vi "Begin.vi"() -> (0 "error out":errorcluster)   [LabVIEW 2013]
doc: "Called before other user functions, this VI is expected to open initial I/O refnums, load in file data, and do all program initialization. Notice that the <B>error out</B> terminal is simply used for data flow. Wiring it to other structures or subVIs ensures that this VI runs first."
uses:
  <vilib>/Rock Robotics/WPI/DriverStation/WPI_DriverStationRobotMode2.ctl
  <vilib>/Rock Robotics/WPI/Joystick/WPI_JoystickDeviceEnum.ctl
  <vilib>/Rock Robotics/WPI/Solenoid/WPI_SolenoidChannel.ctl
  <vilib>/Rock Robotics/WPI/Solenoid/WPI_SolenoidValue.ctl
  Robot Global Data.vi
  <vilib>/Rock Robotics/WPI/Solenoid/WPI_SolenoidOpenDouble.vi
  <vilib>/Rock Robotics/WPI/Solenoid/WPI_SolenoidSetEnum.vi
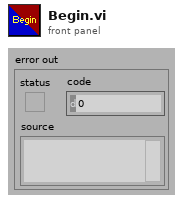
[diagram p1: front panel]
types:
  T1 = typedef "WPI_SolenoidValue.ctl" = enum16{"Off", "On", "Forward", "Reverse"}
  T2 = typedef "WPI_SolenoidChannel.ctl" = enum8{"Solenoid 1", "Solenoid 2", "Solenoid 3", "Solenoid 4", "Solenoid 5", "Solenoid 6", "Solenoid 7", "Solenoid 8", "Invalid"}
  T3 = typedef "WPI_JoystickDeviceEnum.ctl" = enum16{"USB 1", "USB 2", "USB 3", "USB 4", "Kinect 1", "Kinect 2"}
  T4 = typedef "WPI_DriverStationRobotMode2.ctl" = enum16{"Autonomous Disabled", "Autonomous Enabled", "Teleop Disabled", "Teleop Enabled", "Timeout", "Finish", "Test Disabled", "Test Enabled"}
  T5 = typedef "WPI_JoystickDevRef.ctl" = cluster{"Device":T3}
  T6 = typedef "WPI_SolenoidDevRef.ctl" = cluster{"DevStatus":errorcluster, "Solenoid Module":T7, "Forward Solenoid Channel":T2, "Reverse Solenoid Channel":T2}
  T7 = typedef "FPGA_TypedefSolenoidModule.ctl" = enum16{"Solenoid Module 1", "Solenoid Module 2"}
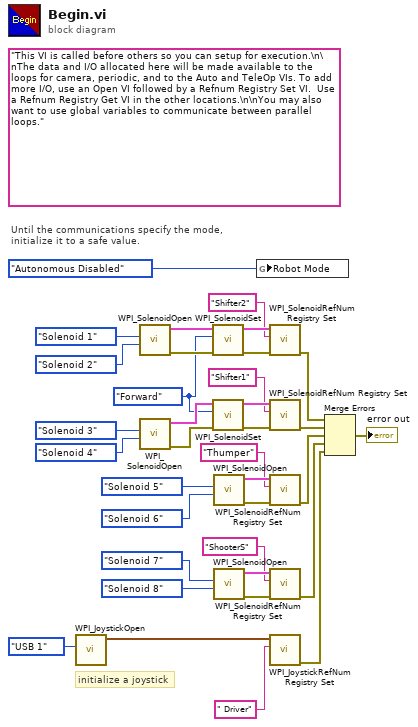
[diagram p0: block diagram]
diagram:
  w7 = WPI_SolenoidValue."Forward" ("Value")
  (unwired) "This VI is called before others so you can setup for execution.\n\nThe data and I/O allocated here will be made available to the loops for camera, periodic, and to the Auto and TeleOp VIs. To add more I/O, use an Open VI followed by a Refnum Registry Set VI.  Use a Refnum Registry Get VI in the other locations.\n\nYou may also want to use global variables to communicate between parallel loops."
  # "initialize a joystick"
  # "Until the communications specify the mode,\ninitialize it to a safe value."
  n1 = call <vilib>:"WPI_JoystickOpen.vi"("JoystickDevice"=WPI_JoystickDeviceEnum."USB 1") -> ("JoystickDevRef"=w6:T5)  [unwired: 10 in]
  n2 = call-poly <vilib>:"WPI_SolenoidOpen.vi"("Reverse Solenoid Channel"=WPI_SolenoidChannel."Solenoid 2", "Forward Solenoid Channel"=WPI_SolenoidChannel."Solenoid 1") -> ("error out"=w18:errorcluster, "SolenoidDevRef"=w19:T6)  [unwired: 8 in]
  n3 = call-poly <vilib>:"WPI_SolenoidOpen.vi"("Reverse Solenoid Channel"=WPI_SolenoidChannel."Solenoid 4", "Forward Solenoid Channel"=WPI_SolenoidChannel."Solenoid 3") -> ("error out"=w11:errorcluster, "SolenoidDevRef"=w12:T6)  [unwired: 8 in]
  n4 = call-poly <vilib>:"WPI_SolenoidSet.vi"("error in (no error)"=w18, "Value"=w7, "SolenoidDevRef"=w19) -> ("error out"=w16:errorcluster, "SolenoidDevRef"=w17:T6)  [unwired: 7 in]
  n5 = call-poly <vilib>:"WPI_SolenoidSet.vi"("error in (no error)"=w11, "Value"=w7, "SolenoidDevRef"=w12) -> ("error out"=w10:errorcluster, "SolenoidDevRef"=w9:T6)  [unwired: 7 in]
  n6 = call-poly <vilib>:"WPI_SolenoidOpen.vi"("Reverse Solenoid Channel"=WPI_SolenoidChannel."Solenoid 6", "Forward Solenoid Channel"=WPI_SolenoidChannel."Solenoid 5") -> ("error out"=w30:errorcluster, "SolenoidDevRef"=w29:T6)  [unwired: 8 in]
  n7 = call-poly <vilib>:"WPI_SolenoidOpen.vi"("Reverse Solenoid Channel"=WPI_SolenoidChannel."Solenoid 8", "Forward Solenoid Channel"=WPI_SolenoidChannel."Solenoid 7") -> ("error out"=w26:errorcluster, "SolenoidDevRef"=w25:T6)  [unwired: 8 in]
  n8 = global write "Robot Global Data.vi" "Robot Mode"(WPI_DriverStationRobotMode2."Autonomous Disabled" ("Robot Mode")) -> ()
  n9 = call <vilib>:"WPI_SolenoidRefNum Registry Set.vi"("error in (no error)"=w16, "refnum name"="Shifter2", "SolenoidDevRef"=w17) -> ("error out"=w1:errorcluster)  [unwired: 7 in, 1 out]
  n10 = call <vilib>:"WPI_SolenoidRefNum Registry Set.vi"("error in (no error)"=w10, "refnum name"="Shifter1", "SolenoidDevRef"=w9) -> ("error out"=w2:errorcluster)  [unwired: 7 in, 1 out]
  n11 = call <vilib>:"WPI_SolenoidRefNum Registry Set.vi"("error in (no error)"=w30, "refnum name"="Thumper", "SolenoidDevRef"=w29) -> ("error out"=w3:errorcluster)  [unwired: 7 in, 1 out]
  n12 = call <vilib>:"WPI_SolenoidRefNum Registry Set.vi"("error in (no error)"=w26, "refnum name"="ShooterS", "SolenoidDevRef"=w25) -> ("error out"=w4:errorcluster)  [unwired: 7 in, 1 out]
  n13 = call <vilib>:"WPI_JoystickRefNum Registry Set.vi"("refnum name"=" Driver", "JoystickDevRef"=w6) -> ("error out"=w5:errorcluster)  [unwired: 8 in, 1 out]
  n14 = Merge Errors(w1, w2, w3, w4, w5) -> (→"error out":errorcluster)
